vi "write_data.vi"(8 "error in (no error)":errorcluster, 10 "data":T1={"n_samples"=1.0}, 11 "Mixture in":refnum<class "Mixture.lvclass">) -> (0 "error out":errorcluster, 3 "Mixture out":refnum<class "Mixture.lvclass">)   [LabVIEW 2020, in "Mixture.lvclass"]
uses:
  Mixture.lvclass
  Controls/mixture_data.ctl
  Mixture.lvclass/Mixture.ctl
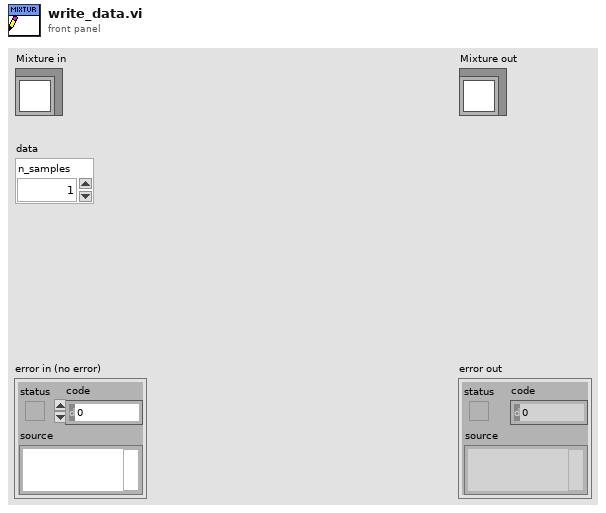
[diagram p1: front panel]
types:
  T1 = typedef "mixture_data.ctl" = cluster{"n_samples":dbl}
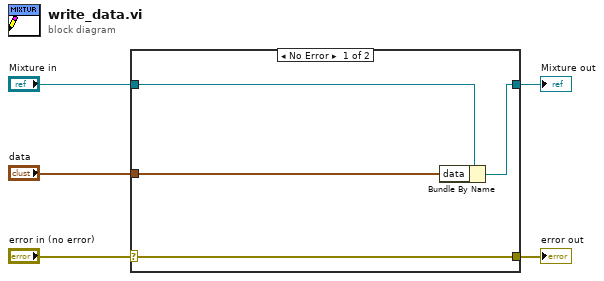
[diagram p0: block diagram]
diagram:
  n1 = case shown="No Error" "error in (no error)" {
    selector: "error in (no error)" -> [w9 w10]
    tunnel: [w9 w10] -> w4
    tunnel: [w7 w11] -> w2
    tunnel: "Mixture in" -> [w8 w11]
    tunnel: "data" -> [w6 _]
    frame No Error {
      n2 = Bundle By Name(cluster=w8, "data"=w6) -> (w7:refnum<class "Mixture.lvclass">)
    }
    frame Error {
    }
  }
  "error out" <- w4
  "Mixture out" <- w2
